vi "Sample 2 - Simple Interaction.vi"() -> ()   [LabVIEW 2016]
panel:
  in  "System Locator":string="usb:ix:0"
  out "Error":errorcluster
  in  "Steps":i32=1000 min=0 max=1000000 step=1
  in  "Amplitude":u32=4000 min=1 max=4000 step=1
  in  "Frequency":u32=8000 min=1 max=18500 step=1
  in  "stop":bool
  in  "Channel":u32
  out "System Index":u32
  in  "forward":bool
  in  "backward":bool
  in  "exit":bool
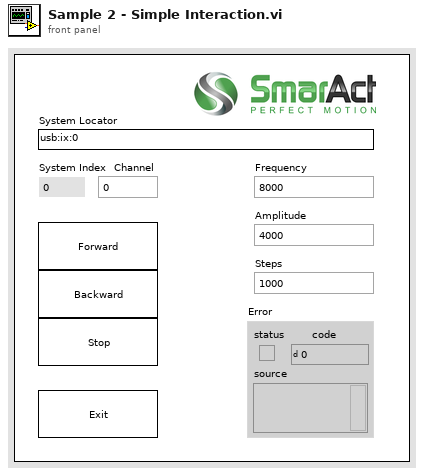
[diagram p1: front panel]
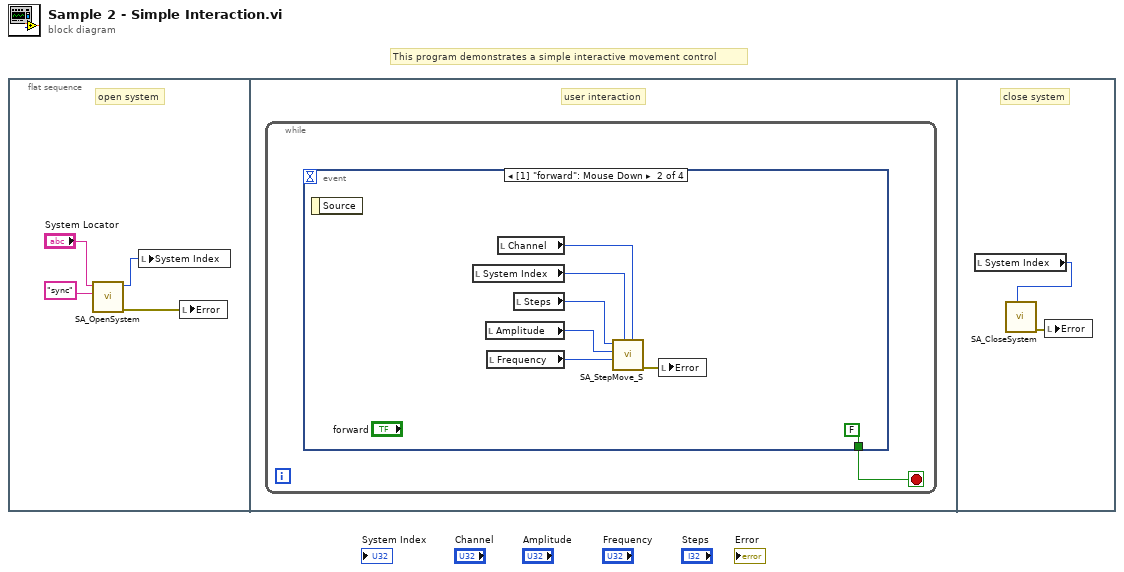
[diagram p0: block diagram]
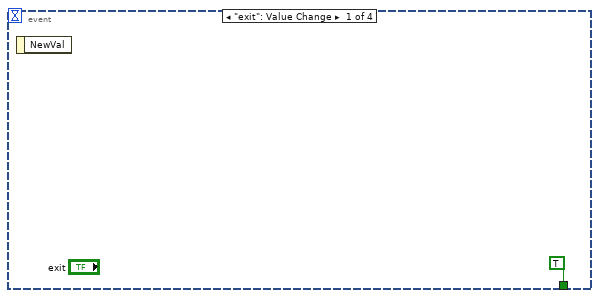
[diagram p2: hidden frame]
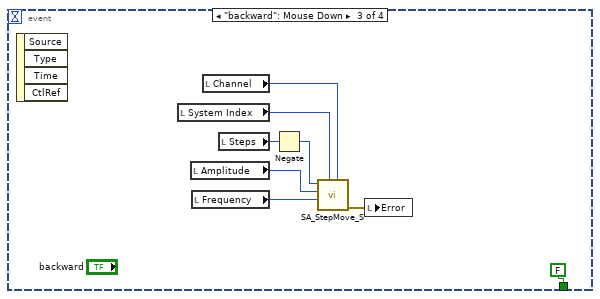
[diagram p3: hidden frame]
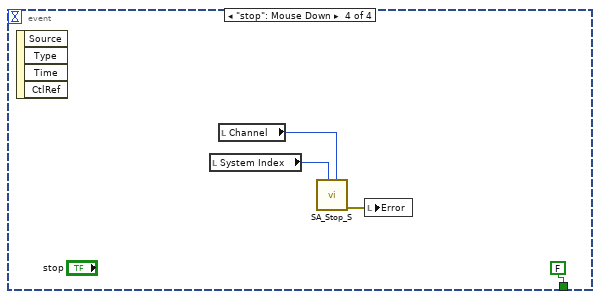
[diagram p4: hidden frame]
diagram:
  # "This program demonstrates a simple interactive movement control"
  n1 = flat-sequence {
    frame #0 {
      # "open system"
      n2 = call <vilib>:"SA_OpenSystem.vi"("options"="sync", "systemLocator"="System Locator") -> ("error out"=w4:errorcluster, "systemIndexOut"=w1:u32)  [unwired: 8 in]
      n3 = local write "System Index"(w1) -> ()
      n4 = local write "Error"(w4) -> ()
    }
    frame #1 {
      # "user interaction"
      n5 = while {
        stop <- w5 stop-if-true
        n6 = event shown="[1] \"forward\": Mouse Down" {
          selector: _ -> [_ _ _ _]
          dyn-events: _ -> [_ _ _ _]
          timeout: _ -> [_ _ _ _]
          tunnel: [TRUE ("exit") FALSE ("exit") FALSE ("exit") FALSE ("exit")] -> w5
          event "exit": Value Change {
            n7 = event-data() -> ()  [unwired: 1 in, 1 out]
          }
          event "forward": Mouse Down {
            n8 = event-data() -> ()  [unwired: 1 in, 1 out]
            n9 = local read "System Index"() -> (w8:u32)
            n10 = local read "Amplitude"() -> (w9:u32)
            n11 = local read "Frequency"() -> (w10:u32)
            n12 = local read "Channel"() -> (w12:u32)
            n13 = local read "Steps"() -> (w11:i32)
            n14 = call <vilib>:"SA_StepMove_S.vi"("channelIndex"=w12, "systemIndex"=w8, "frequency"=w10, "amplitude"=w9, "steps"=w11) -> ("error out"=w7:errorcluster)  [unwired: 6 in]
            n15 = local write "Error"(w7) -> ()
          }
          event "backward": Mouse Down {
            n16 = event-data() -> ()  [unwired: 1 in, 4 out]
            n17 = local read "System Index"() -> (w17:u32)
            n18 = local read "Amplitude"() -> (w18:u32)
            n19 = local read "Frequency"() -> (w19:u32)
            n20 = local read "Channel"() -> (w20:u32)
            n21 = local read "Steps"() -> (w15:i32)
            n22 = Negate(x=w15) -> (-x=w16:i32)
            n23 = call <vilib>:"SA_StepMove_S.vi"("channelIndex"=w20, "systemIndex"=w17, "frequency"=w19, "amplitude"=w18, "steps"=w16) -> ("error out"=w14:errorcluster)  [unwired: 6 in]
            n24 = local write "Error"(w14) -> ()
          }
          event "stop": Mouse Down {
            n25 = event-data() -> ()  [unwired: 1 in, 4 out]
            n26 = local read "System Index"() -> (w23:u32)
            n27 = local read "Channel"() -> (w24:u32)
            n28 = call <vilib>:"SA_Stop_S.vi"("channelIndex"=w24, "systemIndex"=w23) -> ("error out"=w22:errorcluster)  [unwired: 9 in]
            n29 = local write "Error"(w22) -> ()
          }
        }
      }
    }
    frame #2 {
      # "close system"
      n30 = local read "System Index"() -> (w26:u32)
      n31 = call <vilib>:"SA_CloseSystem.vi"("systemIndex"=w26) -> ("error out"=w27:errorcluster)  [unwired: 10 in]
      n32 = local write "Error"(w27) -> ()
    }
  }
